vi "testDMA_9040.vi"() -> ()   [LabVIEW 2020]
uses:
  <vilib>/rvi/Emulation/niFpgaGetClockAttributes.vi
  <vilib>/rvi/Emulation/niFpgaSctlEmulationGetInTimedLoop.vi
  <vilib>/rvi/Emulation/niFpgaEmulationReportErrorSimple.vi
  <vilib>/rvi/DataTransferAndStorage/Container/Common/niFpgaContainerExecOnDevCompGetState.vi
  <vilib>/rvi/Emulation/niFpgaEmulationIsFPGAContextNoSignature.vi
  <vilib>/rvi/errors/niFpgaSetErrorForExecOnDevCompSimple.vi
  <vilib>/rvi/eio/common/nirviEmuReportErrorAndStop.vi
  <vilib>/rvi/DataTransferAndStorage/Container/Common/niFpgaContainerGetUniqueNameForEmu.vi
  <vilib>/rvi/FIFO/Fifo_Resource/nirvififoEmulationSetSize.vi
  <vilib>/rvi/FIFO/Fifo_Resource/nirviFifoEmulationQueueMgr.vi
  <instcachedir>/0/nirviFifoEmulationQueueMgr_E5CAEC123FF24DC58D834DCA3CDAA9B5.lvgen/nirviFifoEmulationQueueMgr_E5CAEC123FF24DC58D834DCA3CDAA9B5_001.vi
  <vilib>/rvi/FIFO/Fifo_Resource/nirvififoEmulationDetermineInputValidOut.vi
  <vilib>/rvi/FIFO/Fifo_Resource/nirvififoEmulationCreateLock.vi
  <vilib>/rvi/Emulation/niFpgaProcessEmulError.vi
  <vilib>/rvi/FIFO/Fifo_Resource/nirvififoEmulationObtainLock.vi
  <vilib>/rvi/FIFO/Fifo_Resource/nirvififoEmulationReleaseLock.vi
  <vilib>/rvi/occurrence/nirviWaitOnOccurrenceBase.vi
  <vilib>/rvi/errors/nirviReportUnexpectedCaseInternalError.vi
  <vilib>/rvi/errors/nirviReportUnexpectedCaseInternalError (U32).vi
  <vilib>/Utility/error.llb/Clear Errors.vi
  <vilib>/rvi/interface/RandomDataEmulation/niFpgaRandomDataHandleErrors.vi
  <vilib>/rvi/eio/common/nirviEmuTemplateMethod_errors.vi
  <vilib>/rvi/Emulation/niFpgaCriticalErrorInLSC.vi
  <vilib>/rvi/DataTransferAndStorage/Container/XNode/niFpgaContainer.xnode
  <vilib>/rvi/FIFO/Fifo_Resource/niFpgaFifoEmulationRefIn.vi
  <vilib>/eio/EIONode/EIONode.xnode
panel:
  out "write back time":u64
  out "tick count elapsed":u32
  out "write DMA timeout count":i16
  in  "number of samples":i16=100
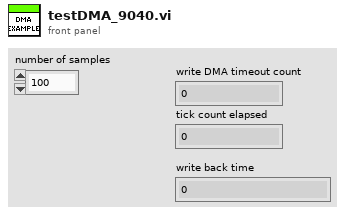
[diagram p1: front panel]
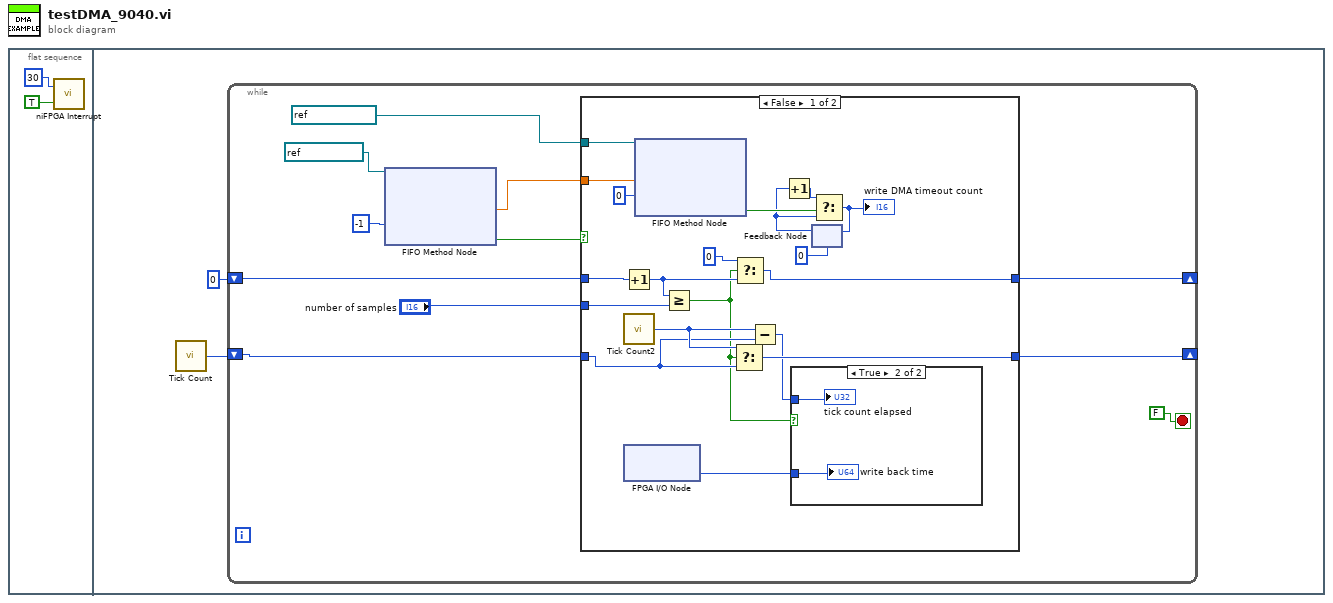
[diagram p0: block diagram]
diagram:
  n1 = flat-sequence {
    frame #0 {
      n2 = call <vilib>:"niFPGA Interrupt.vi"("Wait Until Cleared (F)"=TRUE, "IRQ Number (0)"=u8 30) -> ()  [unwired: 1 in]
    }
    frame #1 {
      n3 = call "Tick Count"() -> ("Tick Count(Ticks)"=w3:u32)
      n4 = while {
        shift-right: [w5] -> _
        shift-left: i16 0 -> [w9]
        shift-right: [w6] -> _
        shift-left: w3 -> [w7]
        stop <- FALSE stop-if-true
        n5 = xnode ("FIFO Method Node")("Timeout"=-1, "FIFO In"=refnum<k21> "Incoming") -> ("Element"=w14:sgl, "Timed Out?"=w10:bool)  [unwired: 1 out]
        n6 = case shown="False" w10 {
          tunnel: refnum<k21> "Outgoing2" ("FIFO In") -> [w34 _]
          tunnel: w14 -> [w33 _]
          tunnel: w9 -> [w32 w38]
          tunnel: "number of samples" -> [w31 _]
          tunnel: w7 -> [w20 w37]
          tunnel: [w30 w37] -> w6
          tunnel: [w27 w38] -> w5
          frame False {
            n7 = Increment(x=w32) -> (x+1=w28:i16)
            n8 = call "Tick Count2"() -> ("Tick Count(Ticks)"=w21:u32)
            n9 = xnode "FPGA I/O Node"() -> ("Time"=w16:u64)  [unwired: 1 in, 1 out]
            n10 = xnode ("FIFO Method Node")("Element"=w33, "Timeout"=0, "FIFO In"=w34) -> ("Timed Out?"=w26:bool)  [unwired: 1 out]
            n11 = Greater Or Equal?(x=w28, y=w31) -> (x >= y?=w19:bool)
            n12 = Select(t=w21, s=w19, f=w20) -> (s? t:f=w30:u32)
            n13 = Select(t=i16 0, s=w19, f=w28) -> (s? t:f=w27:i16)
            n14 = Subtract(x=w21, y=w20) -> (x-y=w18:u32)
            n15 = case shown="True" w19 {
              tunnel: w18 -> [_ w36]
              tunnel: w16 -> [_ w35]
              frame False {
              }
              frame True {
                "tick count elapsed" <- w36
                "write back time" <- w35
              }
            }
            n16 = feedback #1(i16 0) -> (w24:i16)
            n17 = Increment(x=w24) -> (x+1=w23:i16)
            n18 = Select(t=w23, s=w26, f=w24) -> (s? t:f=w22:i16)
            "write DMA timeout count" <- w22
            n19 = feedback-in #1(w22) -> ()
          }
          frame True {
          }
        }
      }
    }
  }
